vi "COMI INT Set Int Chan.vi"(7 "nMode":i32, 9 "nState":i32, 10 "NumCh":i32, 11 "hDevice":u32) -> (2 "function return":i32, 3 "hDevice out":u32)   [LabVIEW 2017, in "Comidll.lvlib"]
doc: "long (COMI_INT_SetIntChan) (HANDLE hDevice, int NumCh, int nState, int nMode);"
uses:
  <userlib>/Comidll/Comidll.lvlib
  <userlib>/Comidll/Comidll.dll
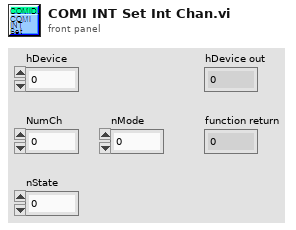
[diagram p1: front panel]
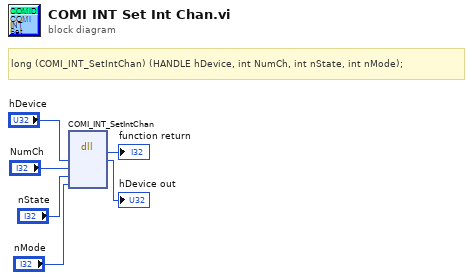
[diagram p0: block diagram]
diagram:
  # "long\t(COMI_INT_SetIntChan) (HANDLE hDevice, int NumCh, int nState, int nMode);"
  n1 = dll-call lib="C:/Program Files/National Instruments/LabVIEW 2017/user.lib/Comidll/Comidll.*" fn="COMI_INT_SetIntChan"("hDevice"="hDevice", "NumCh"="NumCh", "nState"="nState", "nMode"="nMode") -> (→"function return":i32, "hDevice"=→"hDevice out":u32)  [unwired: 6 in, 2 out]
